vi "request.Read formatted request string.vi"(8 "error in (no error)":errorcluster, 11 "Request in":refnum<class "Request.lvclass">) -> (0 "error out":errorcluster, 2 "formatted request string":string, 3 "Request out":refnum<class "Request.lvclass">)   [LabVIEW 2020, in "JSON-RPC Lib.lvlib" / "Request.lvclass"]
uses:
  Request.lvclass
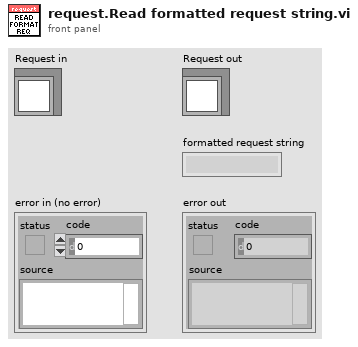
[diagram p1: front panel]
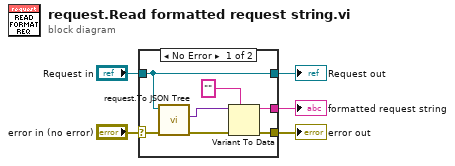
[diagram p0: block diagram]
diagram:
  n1 = case shown="No Error" "error in (no error)" {
    selector: "error in (no error)" -> [w8 w14]
    tunnel: [w9 w14] -> w4
    tunnel: [w12 w13] -> w2
    tunnel: "Request in" -> [w12 w13]
    tunnel: [w10 _] -> w1
    frame No Error {
      n2 = call "request.To JSON Tree.vi"("error in (no error)"=w8, "Request in"=w12) -> ("error out"=w11:errorcluster, "JSON Value out"=w7:variant)  [unwired: 7 in, 1 out]
      n3 = Variant To Data(error in=w11, type="", Variant=w7) -> (data=w10:string, error out=w9:errorcluster)
    }
    frame Error {
    }
  }
  "error out" <- w4
  "Request out" <- w2
  "formatted request string" <- w1
